vi "CheckMemoryLayout.vi"(7 "SrcPointer":T3 {"ImagePointer" format="%.0x"}, 8 "error in":errorcluster, 10 "Format":T1, 11 "DstImage Reference":T2) -> (0 "error out":errorcluster, 2 "Same":bool, 3 "DstImage Reference":T2)   [LabVIEW 2020, in "OpenLvVision_Image.lvlib" / "Management.lvlib"]
uses:
  Management.lvlib
  DataAccess/TypeDef/ImagePointer.ctl
  TypeDef/ImageType.ctl
  TypeDef/Image.ctl
  DataAccess/DataAccess.lvlib
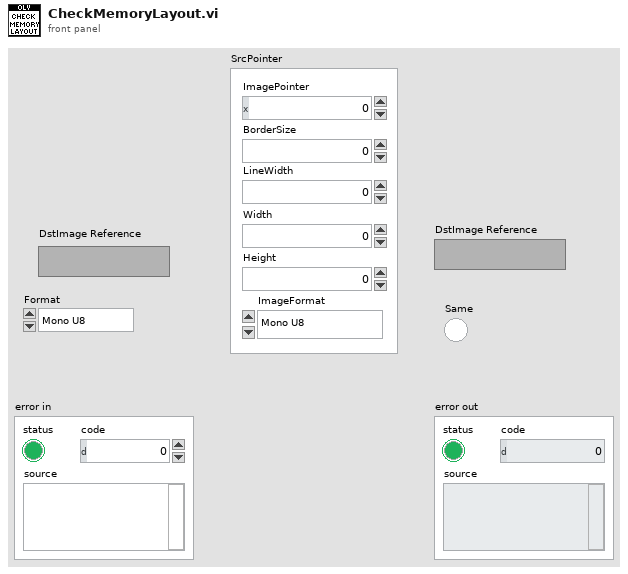
[diagram p1: front panel]
types:
  T1 = typedef "OpenLvVision_Image.lvlib/Management.lvlib/ImageType.ctl" = enum16{"Mono U8", "Mono U16", "Mono I16", "Mono SGL", "Color U32", "Color U64", "Complex CSG"}
  T2 = typedef "OpenLvVision_Image.lvlib/Management.lvlib/Image.ctl" = refnum<image>
  T3 = typedef "OpenLvVision_Image.lvlib/DataAccess.lvlib/ImagePointer.ctl" = cluster{"ImagePointer":u64, "BorderSize":i32, "LineWidth":i32, "Width":i32, "Height":i32, "ImageFormat":T1}
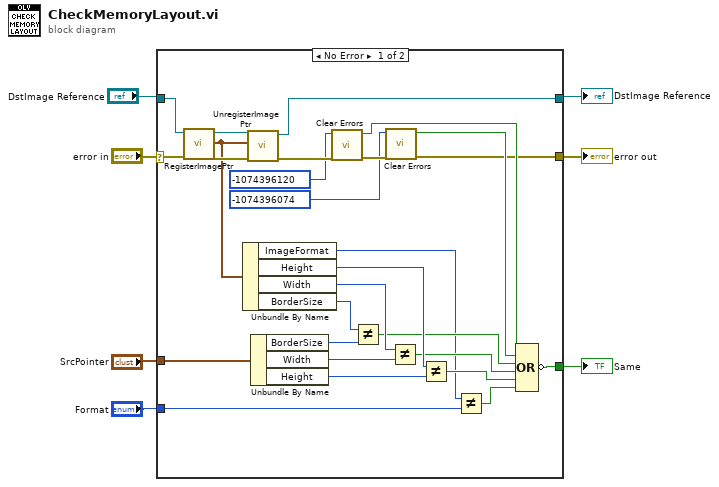
[diagram p0: block diagram]
diagram:
  n1 = case shown="No Error" "error in" {
    selector: "error in" -> [w10 w36]
    tunnel: "DstImage Reference" -> [w34 w35]
    tunnel: [w31 w35] -> w6
    tunnel: "SrcPointer" -> [w29 _]
    tunnel: [w16 _] -> w4
    tunnel: [w11 w36] -> w3
    tunnel: "Format" -> [w9 _]
    frame No Error {
      n2 = call "RegisterImagePtr.vi"("error in"=w10, "Image Reference In"=w34) -> ("error out"=w32:errorcluster, "ImagePointer"=w30:T3, "Image Reference Out"=w33:T2)  [unwired: 7 in]
      n3 = Unbundle By Name(w30) -> ("ImageFormat"=w8:T1, "Height"=w21:i32, "Width"=w22:i32, "BorderSize"=w23:i32)
      n4 = call "UnregisterImagePtr.vi"("error in"=w32, "ImagePointer"=w30, "Image Reference In"=w33) -> ("error out"=w28:errorcluster, "Image Reference Out"=w31:T2)  [unwired: 7 in]
      n5 = Unbundle By Name(w29) -> ("BorderSize"=w26:i32, "Width"=w25:i32, "Height"=w24:i32)
      n6 = call <vilib>:"Clear Errors.vi"("error in (no error)"=w28, "specific error code to clear (0: all)"=-1074396120) -> ("error out"=w15:errorcluster, "specific error cleared?"=w12:bool)  [unwired: 4 in]
      n7 = Not Equal?(x=w23, y=w26) -> (x != y?=w17:bool)
      n8 = call <vilib>:"Clear Errors.vi"("error in (no error)"=w15, "specific error code to clear (0: all)"=-1074396074) -> ("error out"=w11:errorcluster, "specific error cleared?"=w13:bool)  [unwired: 4 in]
      n9 = Not Equal?(x=w22, y=w25) -> (x != y?=w18:bool)
      n10 = Not Equal?(x=w21, y=w24) -> (x != y?=w19:bool)
      n11 = Not Equal?(x=w8, y=w9) -> (x != y?=w20:bool)
      n12 = Compound Arithmetic op=OR(w12, w13, w17, w18, w19, w20) -> (invert w16:bool)
    }
    frame Error {
    }
  }
  "error out" <- w3
  "DstImage Reference" <- w6
  "Same" <- w4
